vi "Manejo de strings.vi"() -> ()   [LabVIEW 2016]
panel:
  out "Nombre Completo":string
  in  "Apellido Materno":string
  in  "Apellido Paterno":string
  in  "Nombre 2":string
  in  "Nombre 1":string
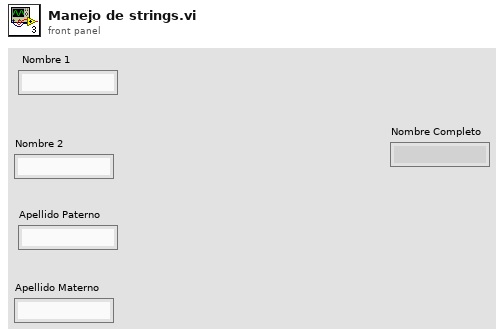
[diagram p1: front panel]
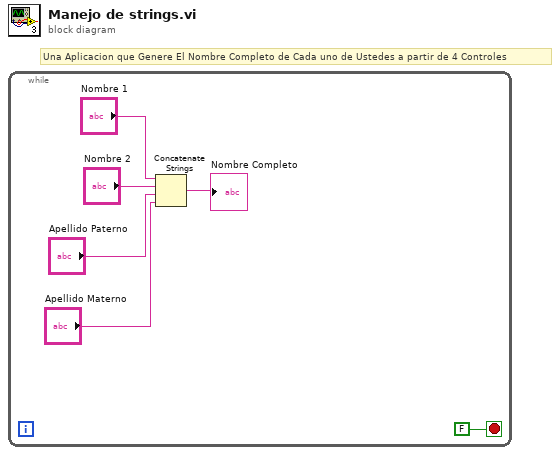
[diagram p0: block diagram]
diagram:
  # "Una Aplicacion que Genere El Nombre Completo de Cada uno de Ustedes a partir de 4 Controles"
  n1 = while {
    stop <- FALSE stop-if-true
    n2 = Concatenate Strings("Nombre 1", "Nombre 2", "Apellido Paterno", "Apellido Materno") -> (→"Nombre Completo":string)
  }
